vi "On Compile - Acyclic Tx - Get Parameters Channels Refs.vi"(8 "error in (no error)":errorcluster, 10 "Channel Data [] In":T3[](array[typedef]) {"Labels Settings"."Label Timestamp Channel Data Reference" format="%.0x"; "Labels Settings"."Label Disable/Trigger Channel Reference" format="%.0x"; "Labels Settings"."Word"."Param Setting"."Item Refs" format="%.0x"; "Labels Settings"."Word"."Param Setting"."Num Bits" min=1 max=32; "Labels Settings"."Word"."Param Setting"."Start Bit" min=8 max=31; "Labels Settings"."Label" format="%.0o"}, 11 "Item Ref In":T1 format="%.0x") -> (0 "error out":errorcluster, 1 "Group":T2 {"VS Refs" format="%.0x"}, 2 "Channel Data [] InOut":T3[](array[typedef]) {"Labels Settings"."Label Timestamp Channel Data Reference" format="%.0x"; "Labels Settings"."Label Disable/Trigger Channel Reference" format="%.0x"; "Labels Settings"."Word"."Param Setting"."Item Refs" format="%.0x"; "Labels Settings"."Word"."Param Setting"."Num Bits" min=1 max=32; "Labels Settings"."Word"."Param Setting"."Start Bit" min=8 max=31; "Labels Settings"."Label" format="%.0o"}, 3 "Item Ref Out":T1 format="%.0x")   [LabVIEW 2019, in "Ballard Arinc-429 System Explorer.lvlib"]
uses:
  Ballard Arinc-429 System Explorer.lvlib
  <vilib>/NI VeriStand/Custom Device API/Custom Device Item Ref.ctl
  Shared/Controls and Global/RT HW Channel.ctl
  Shared/Controls and Global/RT Label Settings.ctl
  Shared/Controls and Global/Label.ctl
  Shared/Controls and Global/transferPeriod.ctl
  Shared/Controls and Global/RT Word Settings.ctl
  Shared/Controls and Global/RT Param Setting.ctl
  Shared/Controls and Global/Start Bit.ctl
  Shared/Controls and Global/Number of Bits.ctl
  <vilib>/NI VeriStand/Custom Device API/Block Data Reference.ctl
  <vilib>/NI VeriStand/Custom Device API/Data Reference.ctl
  Shared/Controls and Global/TransferType.ctl
  <vilib>/NI VeriStand/Custom Device API/Custom Device API.lvlib
  Shared/Ballard Arinc-429 Shared.lvlib
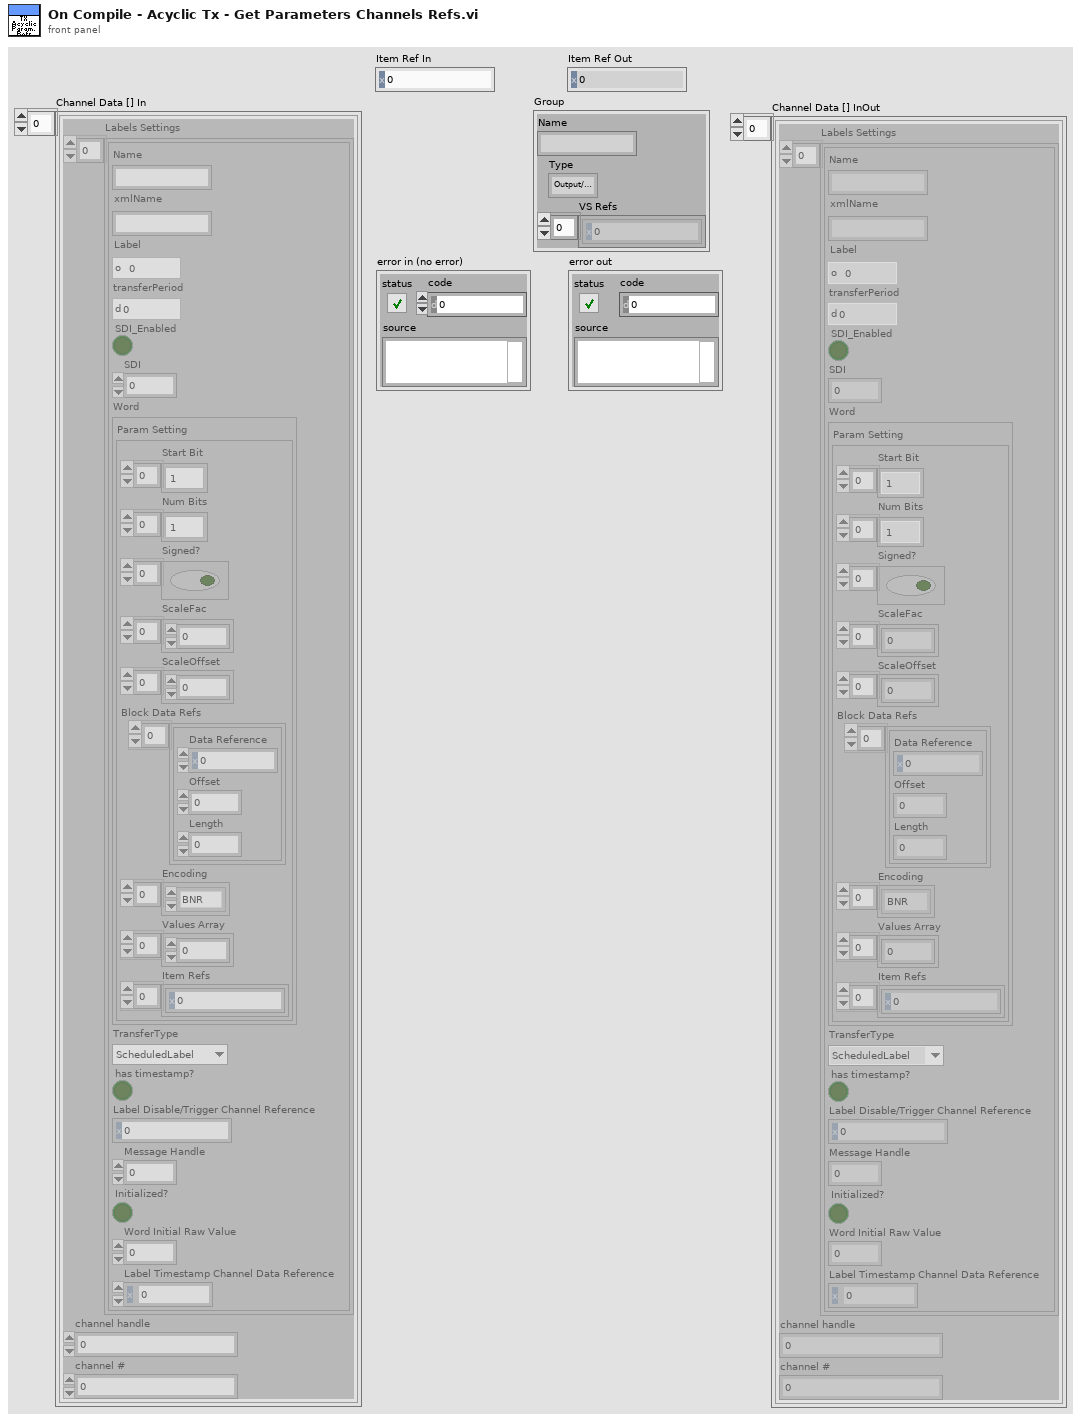
[diagram p1: front panel]
types:
  T1 = typedef "Custom Device API.lvlib/Custom Device Item Ref.ctl" = u64
  T2 = cluster{"Name":string, "Type":enum16{"Output/Write", "Input/Read", "Input/ReadWrite"}, "VS Refs":T1[]}
  T3 = typedef "Ballard Arinc-429 Shared.lvlib/RT HW Channel.ctl" = cluster{"Labels Settings":T4[], "channel handle":u64, "channel #":u16}
  T4 = typedef "Ballard Arinc-429 Shared.lvlib/RT Label Settings.ctl" = cluster{"Name":string, "xmlName":string, "Label":T5, "transferPeriod":T6, "SDI_Enabled":bool, "SDI":u8, "Word":T7, "TransferType":T13, "has timestamp?":bool, "Label Disable/Trigger Channel Reference":T1, "Message Handle":u64, "Initialized?":bool, "Word Initial Raw Value":u32, "Label Timestamp Channel Data Reference":T12}
  T5 = typedef "Ballard Arinc-429 Shared.lvlib/Label.ctl" = u8
  T6 = typedef "Ballard Arinc-429 Shared.lvlib/transferPeriod.ctl" = u32
  T7 = typedef "Ballard Arinc-429 Shared.lvlib/RT Word Settings.ctl" = cluster{"Param Setting":T8}
  T8 = typedef "Ballard Arinc-429 Shared.lvlib/RT Param Setting.ctl" = cluster{"Start Bit":T9[], "Num Bits":T10[], "Signed?":bool[], "ScaleFac":dbl[], "ScaleOffset":dbl[], "Block Data Refs":T11[], "Encoding":enum16{"BNR", "BCD", "Discrete"}[], "Values Array":dbl[], "Item Refs":T1[]}
  T9 = typedef "Ballard Arinc-429 Shared.lvlib/Start Bit.ctl" = i32
  T10 = typedef "Ballard Arinc-429 Shared.lvlib/Number of Bits.ctl" = i32
  T11 = typedef "Custom Device API.lvlib/Block Data Reference.ctl" = cluster{"Data Reference":T12, "Offset":u64, "Length":u64}
  T12 = typedef "Custom Device API.lvlib/Data Reference.ctl" = i32
  T13 = typedef "Ballard Arinc-429 Shared.lvlib/TransferType.ctl" = enum16{"ScheduledLabel", "Acyclic", "Block", "Strobe"}
  T14 = enum16{"Output/Write", "Input/Read", "Input/ReadWrite"}
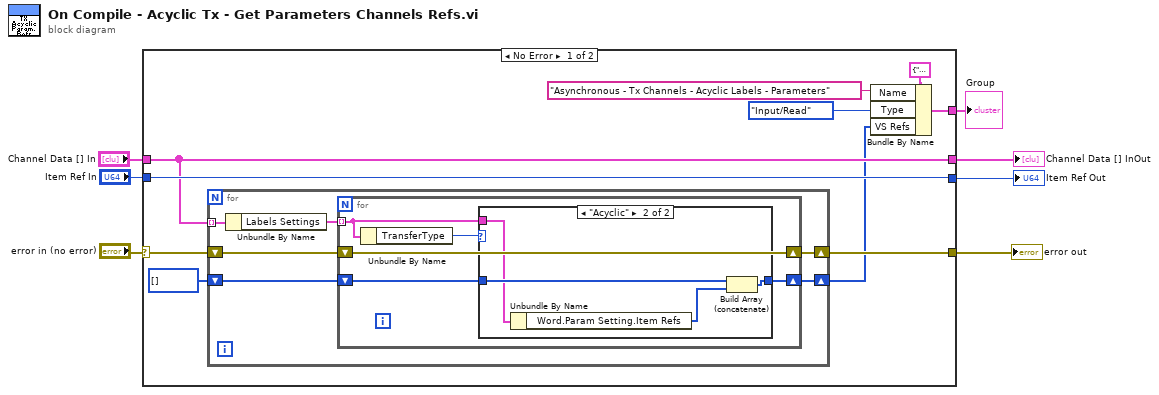
[diagram p0: block diagram]
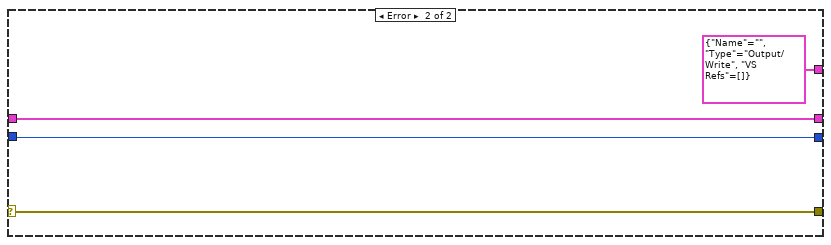
[diagram p3: hidden frame]
diagram:
  n1 = case shown="No Error" "error in (no error)" {
    selector: "error in (no error)" -> [w16 w37]
    tunnel: "Item Ref In" -> [w17 w36]
    tunnel: [w14 w37] -> w5
    tunnel: "Channel Data [] In" -> [w15 w35]
    tunnel: [w15 w35] -> w3
    tunnel: [w17 w36] -> w2
    tunnel: [w9 T2 {"Name"="", "Type"=enum."Output/Write", "VS Refs"=[]} ("Group")] -> w1
    frame No Error {
      n2 = for {
        tunnel: w15 -> [w23] mode=indexing
        shift-right: [w20] -> w14
        shift-left: w16 -> [w22]
        shift-right: [w19] -> w10
        shift-left: T1[] [] -> [w18]
        n3 = Unbundle By Name(w23) -> ("Labels Settings"=w21:T4[])
        n4 = for {
          shift-right: [w28] -> w20
          shift-left: w22 -> [w28]
          tunnel: w21 -> [w25] mode=indexing
          shift-right: [w27] -> w19
          shift-left: w18 -> [w26]
          n5 = Unbundle By Name(w25) -> ("TransferType"=w24:T13)
          n6 = case shown="\"Acyclic\"" w24 {
            tunnel: [w29 w33] -> w27
            tunnel: w26 -> [w29 w32]
            tunnel: w25 -> [_ w30]
            frame Default {
            }
            frame "Acyclic" {
              n7 = Unbundle By Name(w30) -> ("Word.Param Setting.Item Refs"=w31:T1[])
              n8 = Build Array (concatenate)(w32, w31) -> (w33:T1[])
            }
          }
        }
      }
      n9 = Bundle By Name(cluster=T2 {"Name"="", "Type"=enum."Output/Write", "VS Refs"=[]} ("Group"), "Name"="Asynchronous - Tx Channels - Acyclic Labels - Parameters", "Type"=T14."Input/Read", "VS Refs"=w10) -> (w9:T2)
    }
    frame Error {
    }
  }
  "error out" <- w5
  "Item Ref Out" <- w2
  "Channel Data [] InOut" <- w3
  "Group" <- w1
